vi "Status_Ref_API.vi"(0 "DVR In":refnum<data-value>, 11 "Error In":errorcluster) -> (4 "DVR Out":refnum<data-value>, 6 "VI Ref":refnum<vi>, 8 "Status Ref":refnum<vi>, 15 "Error Out":errorcluster)   [LabVIEW 2020, in "Test.lvclass"]
doc: "Status Reference API"
uses:
  Test.lvclass
  Children/INL DNL Test/INL DNL Test.lvclass
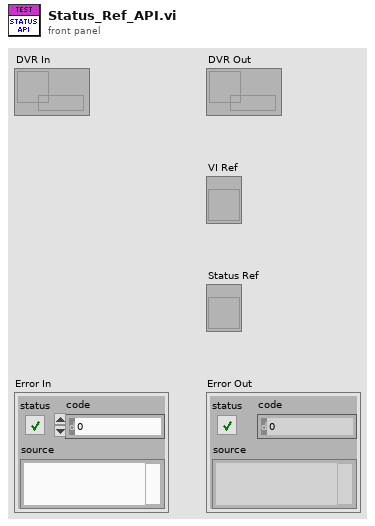
[diagram p1: front panel]
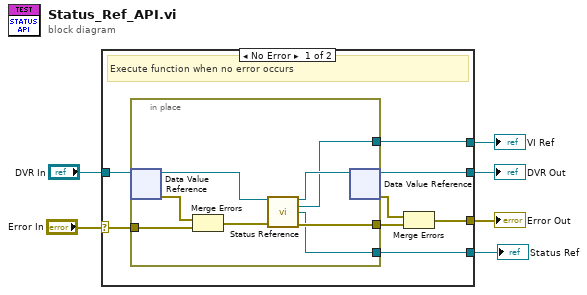
[diagram p0: block diagram]
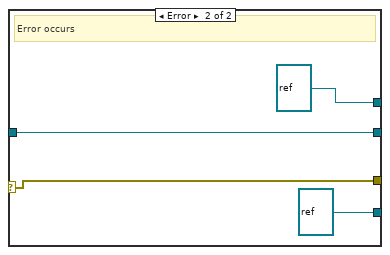
[diagram p2: hidden frame]
diagram:
  n1 = case shown="No Error" "Error In" {
    selector: "Error In" -> [w14 w24]
    tunnel: "DVR In" -> [w13 w25]
    tunnel: [w12 refnum<vi> refnum ("VI ref")] -> w2
    tunnel: [w11 w25] -> w3
    tunnel: [w8 w24] -> w4
    tunnel: [w7 refnum<vi> refnum ("Status Ref")] -> w1
    frame No Error {
      # "Execute function when no error occurs"
      n2 = in-place {
        in-place-border: w14 -> [w22]
        in-place-border: [w17] -> w12
        in-place-border: [w16] -> w9
        in-place-border: [w15] -> w7
        n3 = in-place-dvr #1(w13) -> (w19:refnum<class "Test.lvclass">, w21:errorcluster)
        n4 = Merge Errors(w21, w22) -> (w20:errorcluster)
        n5 = call-dynamic "Status Reference.vi"("Test in"=w19, "Error in"=w20) -> ("Test out"=w18:refnum<class "Test.lvclass">, "VI ref"=w17:refnum<vi>, "Status Ref"=w15:refnum<vi>, "Error out"=w16:errorcluster)  [unwired: 10 in]
        n6 = in-place-dvr #1(w18) -> (w11:refnum<data-value>, w10:errorcluster)
      }
      n7 = Merge Errors(w10, w9) -> (w8:errorcluster)
    }
    frame Error {
      # "Error occurs"
    }
  }
  "Error Out" <- w4
  "DVR Out" <- w3
  "VI Ref" <- w2
  "Status Ref" <- w1
